vi "increase_motor_pow.vi"(0 "delay_per_step":u32, 1 "max_pow":i32) -> ()   [LabVIEW 2017]
uses:
  Untitled Project 6/GlobalVar.vi
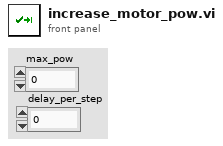
[diagram p1: front panel]
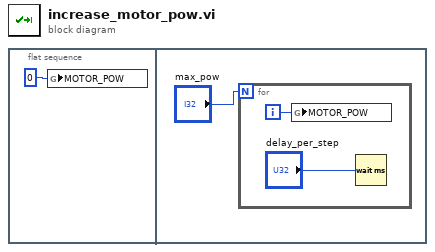
[diagram p0: block diagram]
diagram:
  n1 = flat-sequence {
    frame #0 {
      n2 = global write "GlobalVar.vi" "MOTOR_POW"(i8 0 ("MOTOR_POW")) -> ()
    }
    frame #1 {
      n3 = for {
        N: "max_pow" -> [_]
        i -> [w4]
        n4 = global write "GlobalVar.vi" "MOTOR_POW"(w4) -> ()
        n5 = Wait (ms)(milliseconds to wait="delay_per_step") -> ()  [unwired: 1 out]
      }
    }
  }
